vi "Parse VarINT.vi"(3 "Buffer":u8[](array[numeric]) format="%08b") -> (0 "Numeric":u64 format="%0d", 1 "Bytes":i32)   [LabVIEW 2020, in "Protobuf RAW.lvlib"]
uses:
  Protobuf RAW.lvlib
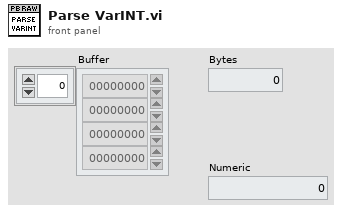
[diagram p1: front panel]
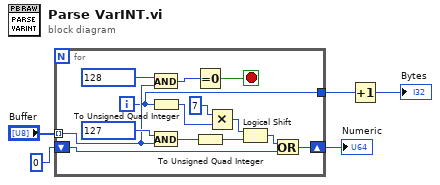
[diagram p0: block diagram]
diagram:
  n1 = for {
    tunnel: "Buffer" -> [w15] mode=indexing
    shift-right: [w13] -> w4
    shift-left: u64 0 -> [w14]
    tunnel: [w9] -> w2
    i -> [w9]
    stop <- w17 stop-if-true
    n2 = And(x=u8 128 ("y"), y=w15) -> (x .and. y?=w18:u8)
    n3 = To Unsigned Quad Integer(1:w9) -> (0:w6:u64)
    n4 = And(x=u8 127 ("y"), y=w15) -> (x .and. y?=w12:u8)
    n5 = Equal To 0?(x=w18) -> (x = 0?=w17:bool)
    n6 = To Unsigned Quad Integer(1:w12) -> (0:w7:u64)
    n7 = Multiply(x=7 ("y"), y=w6) -> (x*y=w8:u64)
    n8 = Logical Shift(y=w8, x=w7) -> (x << y=w11:u64)
    n9 = Or(x=w11, y=w14) -> (x .or. y?=w13:u64)
  }
  "Numeric" <- w4
  n10 = Increment(x=w2) -> (x+1=→"Bytes":i32)
